vi "Assign three values from string to axes.vi"(2 "Queried axes":string[](array[string]), 4 "Input String":string, 5 "error in":errorcluster) -> (10 "Values 3":dbl[](array[numeric]) format="%.6f", 11 "Strings 3":string[](array[string]), 12 "Values 2":dbl[](array[numeric]) format="%.6f", 13 "Strings 2":string[](array[string]), 14 "Values 1":dbl[](array[numeric]) format="%.6f", 15 "Strings 1":string[](array[string]), 16 "Queried axes out":string[](array[string]), 19 "error out":errorcluster)   [LabVIEW 2020]
doc: "This VI assigns three values and/or strings from input string to queried axes. Sub-VI for MVS.vi."
panel:
  # "This vi assigns three values and/or strings from input string to queried axes.  Sub-VI for MVS.vi."
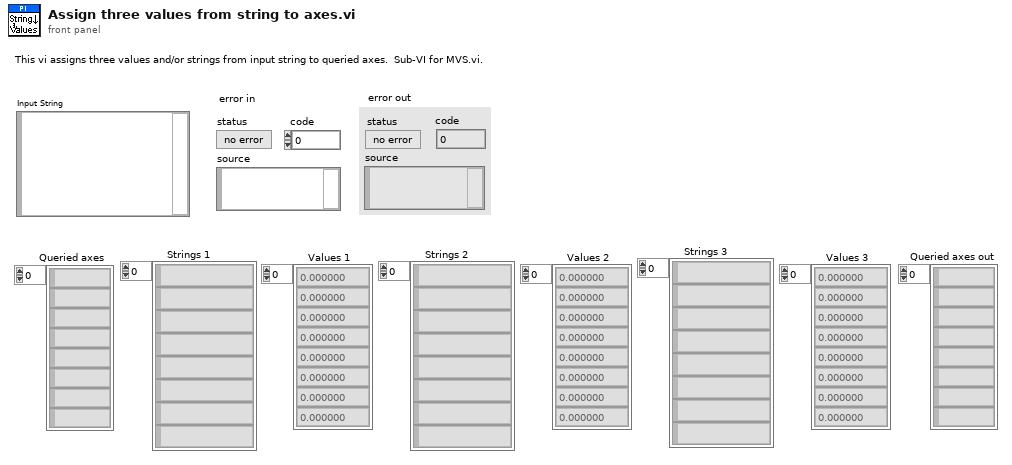
[diagram p1: front panel]
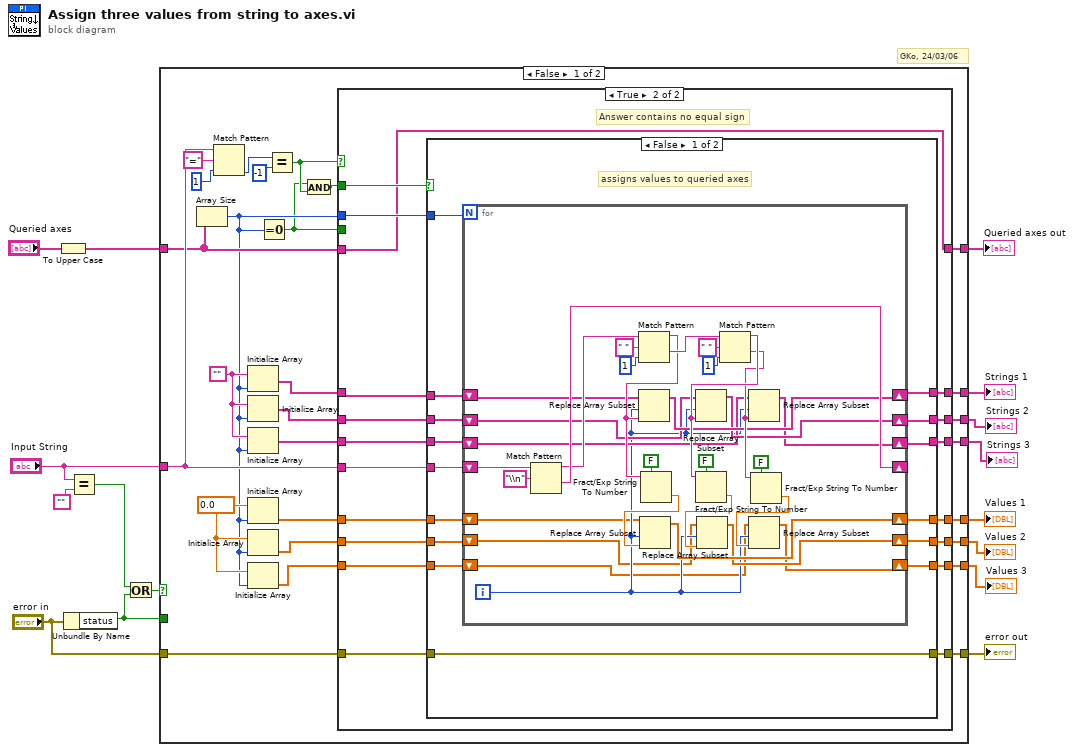
[diagram p0: block diagram]
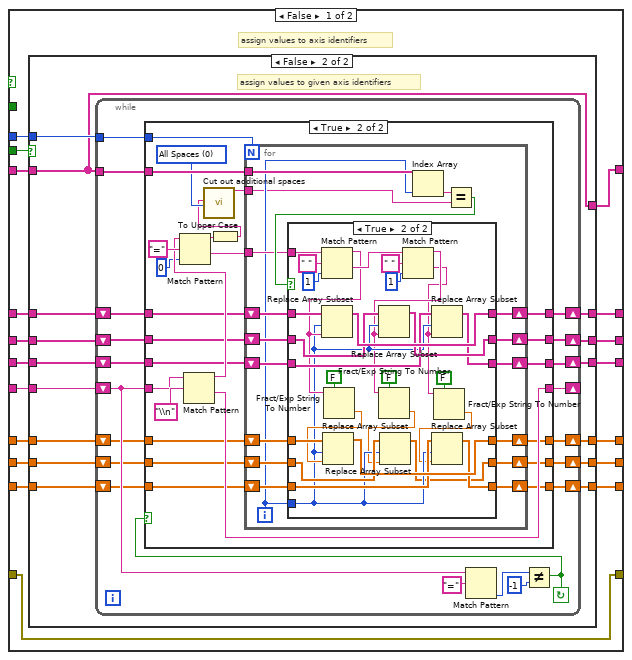
[diagram p2: hidden frame]
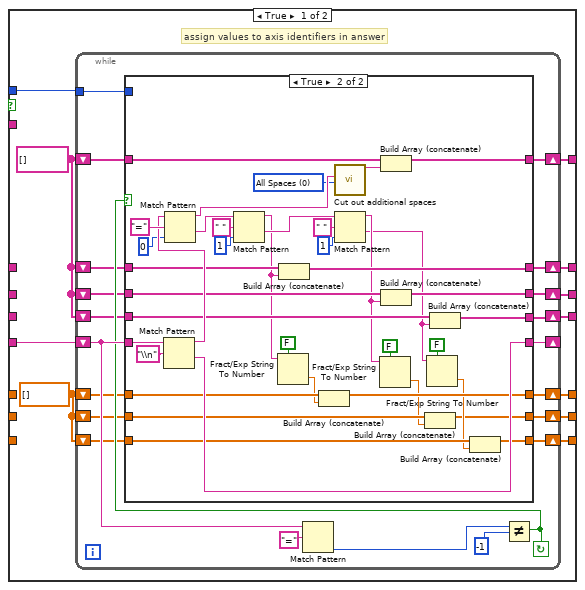
[diagram p3: hidden frame]
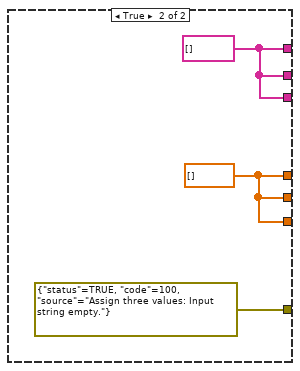
[diagram p7: hidden frame]
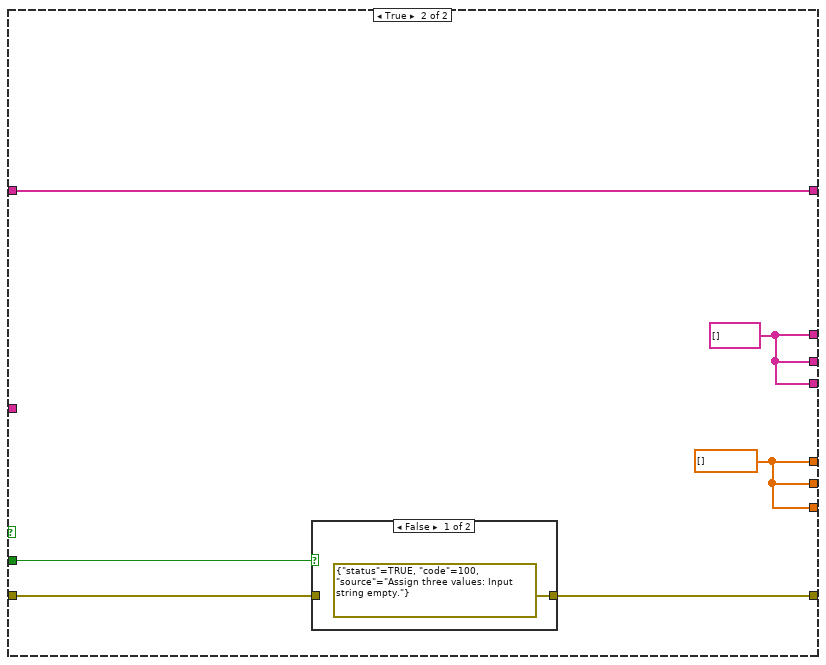
[diagram p8: hidden frame]
diagram:
  # "GKo, 24/03/06"
  n1 = To Upper Case(1:"Queried axes") -> (0:w7:string[])
  n2 = Unbundle By Name("error in") -> ("status"=w9:bool)
  n3 = Equal?(x="Input String", y="") -> (x = y?=w6:bool)
  n4 = Or(x=w6, y=w9) -> (x .or. y?=w11:bool)
  n5 = case shown="False" w11 {
    tunnel: "Input String" -> [w43 _]
    tunnel: [w42 w327] -> w16
    tunnel: w7 -> [w33 w326]
    tunnel: [w31 w330] -> w13
    tunnel: "error in" -> [w30 w331]
    tunnel: [w41 w328] -> w10
    tunnel: w9 -> [_ w329]
    tunnel: [w23 w328] -> w5
    tunnel: [w22 w328] -> w4
    tunnel: [w21 w327] -> w3
    tunnel: [w20 w327] -> w2
    tunnel: [w19 w326] -> w1
    frame False {
      w26 = 0.0 ("Element Data")
      w29 = ""
      n6 = Array Size(array=w33) -> (size(s)=w18:i32)
      n7 = Match Pattern(string=w43, regular expression="=", offset (0)=1) -> (offset past match=w38:i32)  [unwired: 3 out]
      n8 = Initialize Array(w29, w18) -> (w36:string[])
      n9 = Initialize Array(w29, w18) -> (w28:string[])
      n10 = Initialize Array(w29, w18) -> (w27:string[])
      n11 = Initialize Array(w26, w18) -> (w37:dbl[])
      n12 = Initialize Array(w26, w18) -> (w25:dbl[])
      n13 = Initialize Array(w26, w18) -> (w24:dbl[])
      n14 = Equal To 0?(x=w18) -> (x = 0?=w17:bool)
      n15 = Equal?(x=w38, y=-1) -> (x = y?=w34:bool)
      n16 = And(x=w17, y=w34) -> (x .and. y?=w32:bool)
      n17 = case shown="True" w34 {
        tunnel: [w60 w276] -> w42
        tunnel: w43 -> [w61 w275]
        tunnel: w33 -> [w46 w263]
        tunnel: w37 -> [w58 w274]
        tunnel: w18 -> [w59 w273]
        tunnel: w36 -> [w57 w272]
        tunnel: [w56 w271] -> w41
        tunnel: w32 -> [_ w270]
        tunnel: [w55 w269] -> w31
        tunnel: w30 -> [w55 w268]
        tunnel: [w54 w267] -> w23
        tunnel: [w53 w266] -> w22
        tunnel: w28 -> [w52 w262]
        tunnel: w27 -> [w51 w261]
        tunnel: w25 -> [w50 w260]
        tunnel: w24 -> [w49 w259]
        tunnel: [w48 w265] -> w21
        tunnel: [w47 w264] -> w20
        tunnel: [w44 w263] -> w19
        tunnel: w17 -> [w45 _]
        frame False {
          # "assign values to axis identifiers"
          n18 = case shown="False" w45 {
            tunnel: w61 -> [w72 w154]
            tunnel: [w71 w153] -> w60
            tunnel: w59 -> [w70 w152]
            tunnel: w58 -> [_ w151]
            tunnel: w57 -> [_ w150]
            tunnel: [w69 w149] -> w56
            tunnel: [w68 w148] -> w54
            tunnel: [w67 w147] -> w53
            tunnel: w52 -> [_ w146]
            tunnel: w51 -> [_ w145]
            tunnel: w50 -> [_ w144]
            tunnel: w49 -> [_ w143]
            tunnel: [w66 w142] -> w48
            tunnel: [w65 w141] -> w47
            tunnel: w46 -> [_ w140]
            tunnel: [w64 w140] -> w44
            frame True {
              w62 = dbl[] []
              w63 = string[] []
              # "assign values to axis identifiers in answer"
              n19 = while {
                shift-left: w63 -> [w83]
                shift-right: [w84] -> w69
                tunnel: w70 -> [w85]
                shift-left: w62 -> [w87]
                shift-right: [w86] -> w71
                shift-left: w72 -> [w90]
                shift-right: [w89] -> _
                shift-right: [w82] -> w68
                shift-left: w63 -> [w80]
                shift-right: [w81] -> w67
                shift-left: w63 -> [w79]
                shift-right: [w78] -> w66
                shift-left: w62 -> [w76]
                shift-right: [w77] -> w65
                shift-left: w62 -> [w75]
                shift-right: [w74] -> w64
                shift-left: w63 -> [w73]
                stop <- w88 continue-if-true
                n20 = Match Pattern(string=w90, regular expression="=") -> (offset past match=w91:i32)  [unwired: 4 out]
                n21 = Not Equal?(x=w91, y=-1) -> (x != y?=w88:bool)
                n22 = case shown="True" w88 {
                  tunnel: w90 -> [w101 w138]
                  tunnel: [w101 w137] -> w89
                  tunnel: [w100 w109] -> w86
                  tunnel: w87 -> [w100 w110]
                  tunnel: w85 -> [_ _]
                  tunnel: [w99 w118] -> w84
                  tunnel: w83 -> [w99 w119]
                  tunnel: [w98 w116] -> w82
                  tunnel: [w97 w114] -> w81
                  tunnel: w80 -> [w98 w117]
                  tunnel: w79 -> [w97 w115]
                  tunnel: [w96 w102] -> w78
                  tunnel: [w95 w106] -> w77
                  tunnel: w76 -> [w96 w104]
                  tunnel: w75 -> [w95 w107]
                  tunnel: [w94 w131] -> w74
                  tunnel: w73 -> [w94 w120]
                  frame False {
                    # "line contains no equal sign"
                  }
                  frame True {
                    w122 = u16 0 items=["All Spaces", "Only if 1st char.", "Only if last char.", "Only if near \"=\"", "Only if 1st or last char.", "Only multiple"] ("Mode")
                    n23 = Match Pattern(string=w138, regular expression="\\n") -> (before substring=w135:string, after substring=w137:string)  [unwired: 3 out]
                    n24 = Match Pattern(string=w135, regular expression="=", offset (0)=0) -> (before substring=w132:string, after substring=w134:string)  [unwired: 2 out]
                    n25 = Match Pattern(string=w134, regular expression=" ", offset (0)=1) -> (before substring=w113:string, after substring=w126:string)  [unwired: 2 out]
                    n26 = Fract/Exp String To Number(use system decimal point (T)=FALSE, string=w113) -> (number=w108:dbl)  [unwired: 3 out]
                    n27 = Build Array (concatenate)(w119, w113) -> (w118:string[])
                    n28 = Build Array (concatenate)(w110, w108) -> (w109:dbl[])
                    n29 = call "Cut out additional spaces.vi"("String"=w132, "Mode"=w122) -> ("String out"=w121:string)  [unwired: 17 out]
                    n30 = Match Pattern(string=w126, regular expression=" ", offset (0)=1) -> (before substring=w112:string, after substring=w111:string)  [unwired: 2 out]
                    n31 = Fract/Exp String To Number(use system decimal point (T)=FALSE, string=w112) -> (number=w103:dbl)  [unwired: 3 out]
                    n32 = Build Array (concatenate)(w120, w121) -> (w131:string[])
                    n33 = Build Array (concatenate)(w117, w112) -> (w116:string[])
                    n34 = Build Array (concatenate)(w104, w103) -> (w102:dbl[])
                    n35 = Fract/Exp String To Number(use system decimal point (T)=FALSE, string=w111) -> (number=w105:dbl)  [unwired: 3 out]
                    n36 = Build Array (concatenate)(w115, w111) -> (w114:string[])
                    n37 = Build Array (concatenate)(w107, w105) -> (w106:dbl[])
                  }
                }
              }
            }
            frame False {
              # "assign values to given axis identifiers"
              n38 = while {
                shift-left: w150 -> [w163]
                shift-right: [w164] -> w149
                tunnel: w152 -> [w165]
                tunnel: w140 -> [w166]
                shift-left: w151 -> [w168]
                shift-right: [w167] -> w153
                shift-left: w154 -> [w171]
                shift-right: [w170] -> _
                shift-right: [w162] -> w148
                shift-left: w146 -> [w160]
                shift-right: [w161] -> w147
                shift-left: w145 -> [w159]
                shift-right: [w158] -> w142
                shift-left: w144 -> [w156]
                shift-right: [w157] -> w141
                shift-left: w143 -> [w155]
                stop <- w169 continue-if-true
                n39 = Match Pattern(string=w171, regular expression="=") -> (offset past match=w172:i32)  [unwired: 4 out]
                n40 = Not Equal?(x=w172, y=-1) -> (x != y?=w169:bool)
                n41 = case shown="True" w169 {
                  tunnel: w171 -> [w181 w205]
                  tunnel: [w181 w204] -> w170
                  tunnel: [w180 w202] -> w167
                  tunnel: w168 -> [w180 w203]
                  tunnel: w166 -> [_ w199]
                  tunnel: w165 -> [_ w197]
                  tunnel: [w179 w195] -> w164
                  tunnel: w163 -> [w179 w194]
                  tunnel: [w178 w192] -> w162
                  tunnel: [w177 w191] -> w161
                  tunnel: w160 -> [w178 w190]
                  tunnel: w159 -> [w177 w189]
                  tunnel: [w176 w188] -> w158
                  tunnel: [w175 w187] -> w157
                  tunnel: w156 -> [w176 w186]
                  tunnel: w155 -> [w175 w185]
                  frame False {
                  }
                  frame True {
                    w184 = u16 0 items=["All Spaces", "Only if 1st char.", "Only if last char.", "Only if near \"=\"", "Only if 1st or last char.", "Only multiple"] ("Mode")
                    n42 = Match Pattern(string=w205, regular expression="\\n") -> (before substring=w200:string, after substring=w204:string)  [unwired: 3 out]
                    n43 = Match Pattern(string=w200, regular expression="=", offset (0)=0) -> (before substring=w198:string, after substring=w196:string)  [unwired: 2 out]
                    n44 = To Upper Case(1:w198) -> (0:w183:string)
                    n45 = call "Cut out additional spaces.vi"("String"=w183, "Mode"=w184) -> ("String out"=w182:string)  [unwired: 17 out]
                    n46 = for {
                      N: w197 -> [_]
                      shift-right: [w223] -> w202
                      shift-left: w203 -> [w224]
                      tunnel: w199 -> [w222]
                      tunnel: w182 -> [w207]
                      shift-right: [w218] -> w195
                      shift-left: w194 -> [w219]
                      tunnel: w196 -> [w213]
                      shift-right: [w217] -> w192
                      shift-left: w190 -> [w215]
                      shift-right: [w216] -> w191
                      shift-left: w189 -> [w214]
                      shift-right: [w210] -> w188
                      shift-left: w186 -> [w212]
                      shift-right: [w209] -> w187
                      shift-left: w185 -> [w211]
                      i -> [w208]
                      n47 = Index Array(array=w222, index=w208) -> (element=w221:string)
                      n48 = Equal?(x=w221, y=w207) -> (x = y?=w220:bool)
                      n49 = case shown="True" w220 {
                        tunnel: w208 -> [_ w239]
                        tunnel: w224 -> [w230 w258]
                        tunnel: [w230 w257] -> w223
                        tunnel: w219 -> [w229 w256]
                        tunnel: [w229 w255] -> w218
                        tunnel: [w228 w254] -> w217
                        tunnel: [w227 w253] -> w216
                        tunnel: w215 -> [w228 w252]
                        tunnel: w214 -> [w227 w251]
                        tunnel: w213 -> [_ w250]
                        tunnel: w212 -> [w226 w241]
                        tunnel: w211 -> [w225 w240]
                        tunnel: [w226 w237] -> w210
                        tunnel: [w225 w238] -> w209
                        frame False {
                        }
                        frame True {
                          n50 = Match Pattern(string=w250, regular expression=" ", offset (0)=1) -> (before substring=w243:string, after substring=w245:string)  [unwired: 2 out]
                          n51 = Replace Array Subset(array=w256, new element=w243, index=w239) -> (w255:string[])
                          n52 = Fract/Exp String To Number(use system decimal point (T)=FALSE, string=w243) -> (number=w242:dbl)  [unwired: 3 out]
                          n53 = Replace Array Subset(array=w258, new element=w242, index=w239) -> (w257:dbl[])
                          n54 = Match Pattern(string=w245, regular expression=" ", offset (0)=1) -> (before substring=w234:string, after substring=w231:string)  [unwired: 2 out]
                          n55 = Replace Array Subset(array=w252, new element=w234, index=w239) -> (w254:string[])
                          n56 = Fract/Exp String To Number(use system decimal point (T)=FALSE, string=w234) -> (number=w233:dbl)  [unwired: 3 out]
                          n57 = Replace Array Subset(array=w241, new element=w233, index=w239) -> (w237:dbl[])
                          n58 = Replace Array Subset(array=w251, new element=w231, index=w239) -> (w253:string[])
                          n59 = Fract/Exp String To Number(use system decimal point (T)=FALSE, string=w231) -> (number=w232:dbl)  [unwired: 3 out]
                          n60 = Replace Array Subset(array=w240, new element=w232, index=w239) -> (w238:dbl[])
                        }
                      }
                    }
                  }
                }
              }
            }
          }
        }
        frame True {
          # "Answer contains no equal sign"
          n61 = case shown="False" w270 {
            tunnel: [w291 w323] -> w276
            tunnel: w275 -> [w290 _]
            tunnel: w274 -> [w289 _]
            tunnel: w273 -> [w288 _]
            tunnel: w272 -> [w285 _]
            tunnel: [w287 w324] -> w271
            tunnel: [w286 errorcluster {"status"=TRUE, "code"=100, "source"="Assign three values: Input string empty."} ("error out")] -> w269
            tunnel: w268 -> [w286 _]
            tunnel: [w278 w324] -> w267
            tunnel: [w277 w324] -> w266
            tunnel: [w280 w323] -> w265
            tunnel: [w279 w323] -> w264
            tunnel: w262 -> [w284 _]
            tunnel: w261 -> [w283 _]
            tunnel: w260 -> [w282 _]
            tunnel: w259 -> [w281 _]
            frame False {
              # "assigns values to queried axes"
              n62 = for {
                N: w288 -> [_]
                shift-right: [w300] -> w291
                shift-left: w289 -> [w294]
                shift-right: [w321] -> _
                shift-left: w290 -> [w322]
                shift-right: [w303] -> w287
                shift-left: w285 -> [w304]
                shift-right: [w302] -> w278
                shift-left: w284 -> [w296]
                shift-right: [w301] -> w277
                shift-left: w283 -> [w297]
                shift-right: [w299] -> w280
                shift-left: w282 -> [w293]
                shift-right: [w298] -> w279
                shift-left: w281 -> [w292]
                i -> [w295]
                n63 = Match Pattern(string=w322, regular expression="\\n") -> (before substring=w305:string, after substring=w321:string)  [unwired: 3 out]
                n64 = Match Pattern(string=w305, regular expression=" ", offset (0)=1) -> (before substring=w313:string, after substring=w315:string)  [unwired: 2 out]
                n65 = Replace Array Subset(array=w304, new element=w313, index=w295) -> (w303:string[])
                n66 = Fract/Exp String To Number(use system decimal point (T)=FALSE, string=w313) -> (number=w312:dbl)  [unwired: 3 out]
                n67 = Replace Array Subset(array=w294, new element=w312, index=w295) -> (w300:dbl[])
                n68 = Match Pattern(string=w315, regular expression=" ", offset (0)=1) -> (before substring=w309:string, after substring=w306:string)  [unwired: 2 out]
                n69 = Replace Array Subset(array=w296, new element=w309, index=w295) -> (w302:string[])
                n70 = Fract/Exp String To Number(use system decimal point (T)=FALSE, string=w309) -> (number=w308:dbl)  [unwired: 3 out]
                n71 = Replace Array Subset(array=w293, new element=w308, index=w295) -> (w299:dbl[])
                n72 = Replace Array Subset(array=w297, new element=w306, index=w295) -> (w301:string[])
                n73 = Fract/Exp String To Number(use system decimal point (T)=FALSE, string=w306) -> (number=w307:dbl)  [unwired: 3 out]
                n74 = Replace Array Subset(array=w292, new element=w307, index=w295) -> (w298:dbl[])
              }
            }
            frame True {
              w323 = dbl[] []
              w324 = string[] []
            }
          }
        }
      }
    }
    frame True {
      w328 = string[] []
      w327 = dbl[] [] ("Step Size")
      # "Error"
      n75 = case shown="False" w329 {
        tunnel: w331 -> [_ w333]
        tunnel: [errorcluster {"status"=TRUE, "code"=100, "source"="Assign three values: Input string empty."} ("error out") w333] -> w330
        frame False {
        }
        frame True {
        }
      }
    }
  }
  "Values 1" <- w16
  "error out" <- w13
  "Strings 1" <- w10
  "Strings 2" <- w5
  "Values 2" <- w3
  "Strings 3" <- w4
  "Values 3" <- w2
  "Queried axes out" <- w1
